vi "Enum Data Update.vi"(8 "error in (no error)":errorcluster, 10 "Value":string, 11 "Enum in":refnum<vi>) -> (0 "error out":errorcluster, 3 "Enum out":refnum<vi>)   [LabVIEW 2021]
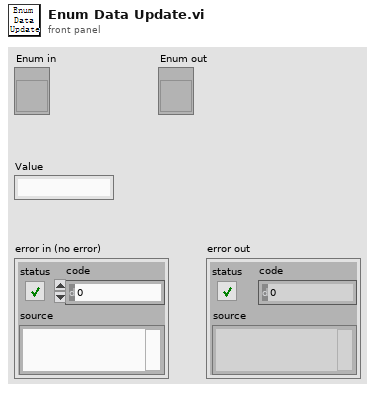
[diagram p1: front panel]
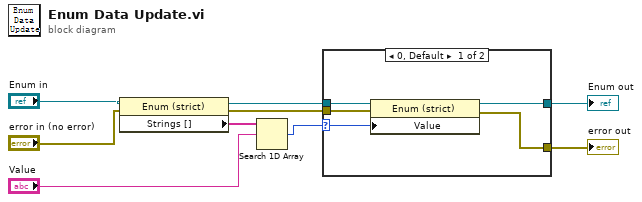
[diagram p0: block diagram]
diagram:
  n1 = property class="Enum (strict)"(reference="Enum in", error in="error in (no error)") -> (reference out=w8:refnum<vi>, error out=w4:errorcluster, "Strings []"=w5:string[])
  n2 = Search 1D Array(1D array=w5, element="Value") -> (index of element=w1:i32)  [unwired: 1 in]
  n3 = case shown="0, Default" w1 {
    selector: w1 -> [w10 _]
    tunnel: [w14 w16] -> w9
    tunnel: w8 -> [w13 w16]
    tunnel: w4 -> [w12 w15]
    tunnel: [w11 w15] -> w2
    frame 0, Default {
      n4 = property class="Enum (strict)"(reference=w13, error in=w12, "Value"=w10) -> (reference out=w14:refnum<vi>, error out=w11:errorcluster)
    }
    frame -1 {
    }
  }
  "Enum out" <- w9
  "error out" <- w2
